vi "CAN output.vi"(4 "error in (no error)":errorcluster, 7 "CANopen in":refnum<class "CANopen.lvclass">) -> (0 "error out":errorcluster, 2 "Output image":u8[](array[numeric]), 3 "CANopen out":refnum<class "CANopen.lvclass">)   [LabVIEW 2024, in "canopen.lvlib" / "CANopen.lvclass"]
doc: "Returns a copy of the internally owned output image. This does not trigger any action: it merely returns the *actual* status of the outputs."
uses:
  CANopen.lvclass
  CANopen.lvclass/CANopen.ctl
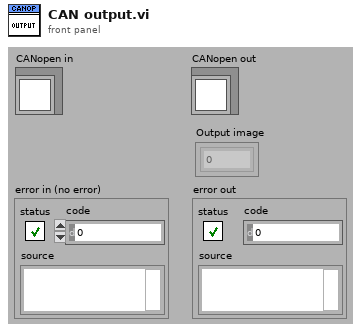
[diagram p1: front panel]
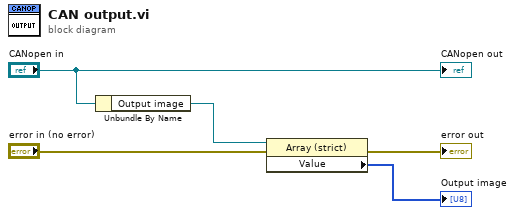
[diagram p0: block diagram]
diagram:
  n1 = Unbundle By Name("CANopen in") -> ("Output image"=w4:refnum<vi>)
  n2 = property class="Array (strict)"(reference=w4, error in="error in (no error)") -> (error out=→"error out":errorcluster, "Value"=→"Output image":u8[])  [unwired: 1 out]
  "CANopen out" <- "CANopen in"
